vi "Write Standad Header.vi"(8 "error in (no error)":errorcluster, 11 "Save Image in":refnum<class "Save Image.lvclass">) -> (0 "error out":errorcluster, 3 "Save Image out":refnum<class "Save Image.lvclass">)   [LabVIEW 2018, in "Save Image.lvclass"]
uses:
  Save Image.lvclass
  <userlib>/gfitsio/gfitsio-write-key-string.vi
  <userlib>/gfitsio/gfitsio-write-key-integer.vi
  <userlib>/gfitsio/gfitsio-write-key-double.vi
  <userlib>/gfitsio/gfitsio.lvlib
  Simulated_Header/Simulated_Header.lvclass
  <vilib>/Utility/Data Type/NI_Data Type.lvlib
panel:
  out "Header Content":T1
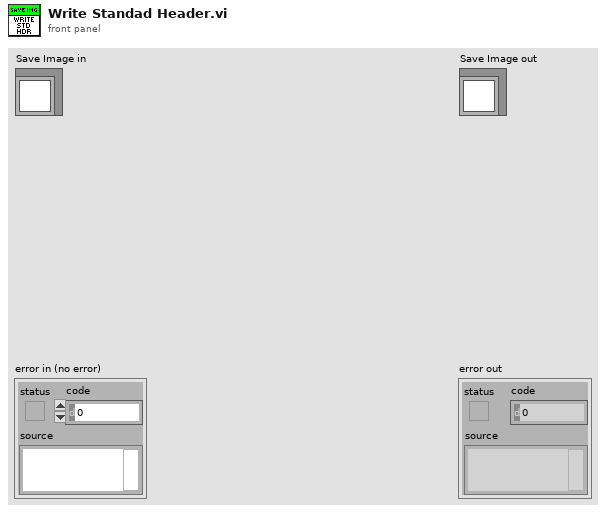
[diagram p1: front panel]
types:
  T1 = cluster{"FILENAME":cluster{"Name":string, "Value":string, "Comment":string}, "OBSERVER":cluster{"Name":string, "Value":string, "Comment":string}, "PROGRID":cluster{"Name":string, "Value":string, "Comment":string}, "OBJECT":cluster{"Name":string, "Value":string, "Comment":string}, "NIGHTDIR":cluster{"Name":string, "Value":string, "Comment":string}, "CHANNEL":cluster{"Name":string, "Value":string, "Comment":string}, "INSTRUME":cluster{"Name":string, "Value":string, "Comment":string}, "NEXPSEQ":cluster{"Name":string, "Value":u16, "Comment":string}, "SEQINDEX":cluster{"Name":string, "Value":u16, "Comment":string}, "OBSTYPE":cluster{"Name":string, "Value":string, "Comment":string}, "READMOD":cluster{"Name":string, "Value":string, "Comment":string}, "READMODE":cluster{"Name":string, "Value":string, "Comment":string}, "ACQMODE":cluster{"Name":string, "Value":string, "Comment":string}, "PREAMP":cluster{"Name":string, "Value":string, "Comment":string}, "READOUT":cluster{"Name":string, "Value":string, "Comment":string}, "VSHIFT":cluster{"Name":string, "Value":string, "Comment":string}, "TRIGGER":cluster{"Name":string, "Value":string, "Comment":string}, "EMMODE":cluster{"Name":string, "Value":string, "Comment":string}, "EMGAIN":cluster{"Name":string, "Value":u16, "Comment":string}, "VBIN":cluster{"Name":string, "Value":u16, "Comment":string}, "HBIN":cluster{"Name":string, "Value":u16, "Comment":string}, "INITLIN":cluster{"Name":string, "Value":u16, "Comment":string}, "INITCOL":cluster{"Name":string, "Value":u16, "Comment":string}, "FINALLIN":cluster{"Name":string, "Value":u16, "Comment":string}, "FINALCOL":cluster{"Name":string, "Value":u16, "Comment":string}, "KSERLEN":cluster{"Name":string, "Value":u16, "Comment":string}, "SHUTTER":cluster{"Name":string, "Value":string, "Comment":string}, "OPENSHT":cluster{"Name":string, "Value":u16, "Comment":string}, "CLOSESHT":cluster{"Name":string, "Value":u16, "Comment":string}, "DATE":cluster{"Name":string, "Value":string, "Comment":string}, "GAIN":cluster{"Name":string, "Value":dbl, "Comment":string}, "GAINERR":cluster{"Name":string, "Value":dbl, "Comment":string}, "RDNOISE":cluster{"Name":string, "Value":dbl, "Comment":string}, "RNOISERR":cluster{"Name":string, "Value":dbl, "Comment":string}, "SKYFIBER":cluster{"Name":string, "Value":string, "Comment":string}, "CALFIBER":cluster{"Name":string, "Value":string, "Comment":string}, "UTDATE":cluster{"Name":string, "Value":string, "Comment":string}, "LOCTIME":cluster{"Name":string, "Value":string, "Comment":string}, "MJD":cluster{"Name":string, "Value":dbl, "Comment":string}, "OBSLON":cluster{"Name":string, "Value":string, "Comment":string}, "OBSLAT":cluster{"Name":string, "Value":string, "Comment":string}, "OBSALT":cluster{"Name":string, "Value":dbl, "Comment":string}, "EXPTIME":cluster{"Name":string, "Value":dbl, "Comment":string}, "TELRA":cluster{"Name":string, "Value":string, "Comment":string}, "TELDEC":cluster{"Name":string, "Value":string, "Comment":string}, "RA":cluster{"Name":string, "Value":string, "Comment":string}, "DEC":cluster{"Name":string, "Value":string, "Comment":string}, "RA_DEG":cluster{"Name":string, "Value":dbl, "Comment":string}, "DEC_DEG":cluster{"Name":string, "Value":dbl, "Comment":string}, "EPOCH":cluster{"Name":string, "Value":dbl, "Comment":string}, "HA":cluster{"Name":string, "Value":string, "Comment":string}, "HAD":cluster{"Name":string, "Value":dbl, "Comment":string}, "AIRMASS":cluster{"Name":string, "Value":dbl, "Comment":string}, "AMSTART":cluster{"Name":string, "Value":dbl, "Comment":string}, "AMEND":cluster{"Name":string, "Value":dbl, "Comment":string}, "XOFFSET":cluster{"Name":string, "Value":dbl, "Comment":string}, "YOFFSET":cluster{"Name":string, "Value":dbl, "Comment":string}, "PA":cluster{"Name":string, "Value":dbl, "Comment":string}, "CAMFOC":cluster{"Name":string, "Value":string, "Comment":string}, "TELFOC":cluster{"Name":string, "Value":dbl, "Comment":string}, "TCSUT":cluster{"Name":string, "Value":string, "Comment":string}, "TCSST":cluster{"Name":string, "Value":string, "Comment":string}, "MOONDIST":cluster{"Name":string, "Value":dbl, "Comment":string}, "MOONALT":cluster{"Name":string, "Value":dbl, "Comment":string}, "MOONPHAS":cluster{"Name":string, "Value":string, "Comment":string}, "ADC":cluster{"Name":string, "Value":string, "Comment":string}, "ADCSPEED":cluster{"Name":string, "Value":dbl, "Comment":string}, "CALMIRR":cluster{"Name":string, "Value":string, "Comment":string}, "GUIDING":cluster{"Name":string, "Value":string, "Comment":string}, "GUIDTEXP":cluster{"Name":string, "Value":dbl, "Comment":string}, "GUIDFREQ":cluster{"Name":string, "Value":dbl, "Comment":string}, "GUIDOBJX":cluster{"Name":string, "Value":dbl, "Comment":string}, "GUIDOBJY":cluster{"Name":string, "Value":dbl, "Comment":string}, "AVGYCORR":cluster{"Name":string, "Value":dbl, "Comment":string}, "AVGXCORR":cluster{"Name":string, "Value":dbl, "Comment":string}, "GFOCUS":cluster{"Name":string, "Value":dbl, "Comment":string}, "THARLAMP":cluster{"Name":string, "Value":string, "Comment":string}, "HALLAMP":cluster{"Name":string, "Value":string, "Comment":string}, "AGITATOR":cluster{"Name":string, "Value":string, "Comment":string}, "THARMIRR":cluster{"Name":string, "Value":string, "Comment":string}, "DSTATUS":cluster{"Name":string, "Value":string, "Comment":string}, "DPOS":cluster{"Name":string, "Value":dbl, "Comment":string}, "DTEMP":cluster{"Name":string, "Value":dbl, "Comment":string}, "DHUM":cluster{"Name":string, "Value":string, "Comment":string}, "DLAMP":cluster{"Name":string, "Value":string, "Comment":string}, "DFLAT":cluster{"Name":string, "Value":string, "Comment":string}, "TEMPEXT":cluster{"Name":string, "Value":string, "Comment":string}, "PRESSURE":cluster{"Name":string, "Value":string, "Comment":string}, "HUMIDITY":cluster{"Name":string, "Value":string, "Comment":string}, "WINDDIR":cluster{"Name":string, "Value":string, "Comment":string}, "WINSPEED":cluster{"Name":string, "Value":dbl, "Comment":string}, "SHTTTL":cluster{"Name":string, "Value":string, "Comment":string}, "COOLER":cluster{"Name":string, "Value":string, "Comment":string}, "TEMP":cluster{"Name":string, "Value":u16, "Comment":string}, "TEMPST":cluster{"Name":string, "Value":string, "Comment":string}, "SERN":cluster{"Name":string, "Value":u16, "Comment":string}, "COMMENT":cluster{"Name":string, "Value":string, "Comment":string}, "SIMPLE":cluster{"Name":string, "Value":string, "Comment":string}, "BITPIX":cluster{"Name":string, "Value":u16, "Comment":string}, "NAXIS":cluster{"Name":string, "Value":u16, "Comment":string}, "EXTEND":cluster{"Name":string, "Value":string, "Comment":string}, "FRAME_T":cluster{"Name":string, "Value":string, "Comment":string}, "VCLOCK":cluster{"Name":string, "Value":string, "Comment":string}, "ADCHNNL":cluster{"Name":string, "Value":u16, "Comment":string}, "JD":cluster{"Name":string, "Value":dbl, "Comment":string}, "SD":cluster{"Name":string, "Value":string, "Comment":string}}
  T2 = cluster{"Name":string, "Value":string, "Comment":string}
  T3 = cluster{"Name":string, "Value":u16, "Comment":string}
  T4 = typedef "NI_Data Type.lvlib/Data Type.ctl" = enum8{"Invalid Type", "Void", "I8", "I16", "I32", "I64", "U8", "U16", "U32", "U64", "Single Float", "Double Float", "Extended Float", "Single Complex", "Double Complex", "Extended Complex", "Enum U8", "Enum U16", "Enum U32", "Enum U64", "Single Float With Unit", "Double Float With Unit", "Extended Float With Unit", "Single Complex with Unit", "Double Complex with Unit", "Extended Complex with Unit", "Boolean", "String", "Path", "Picture", "Tag", "Array", "Cluster", "Variant", "LV Variant", "Waveform", "Timestamp", "Digital Waveform", "Digital Data", "ExpressData", "Refnum", "External Data", "VI", "Poly VI", "LabVIEW Class Instance", "Fixed Point"}
  T5 = cluster{"Name":string, "Value":i32, "Comment":string}
  T6 = cluster{"Name":string, "Value":dbl, "Comment":string}
  T7 = typedef "gfitsio.lvlib/gfitsio-refnum.ctl" = refnum<k1>
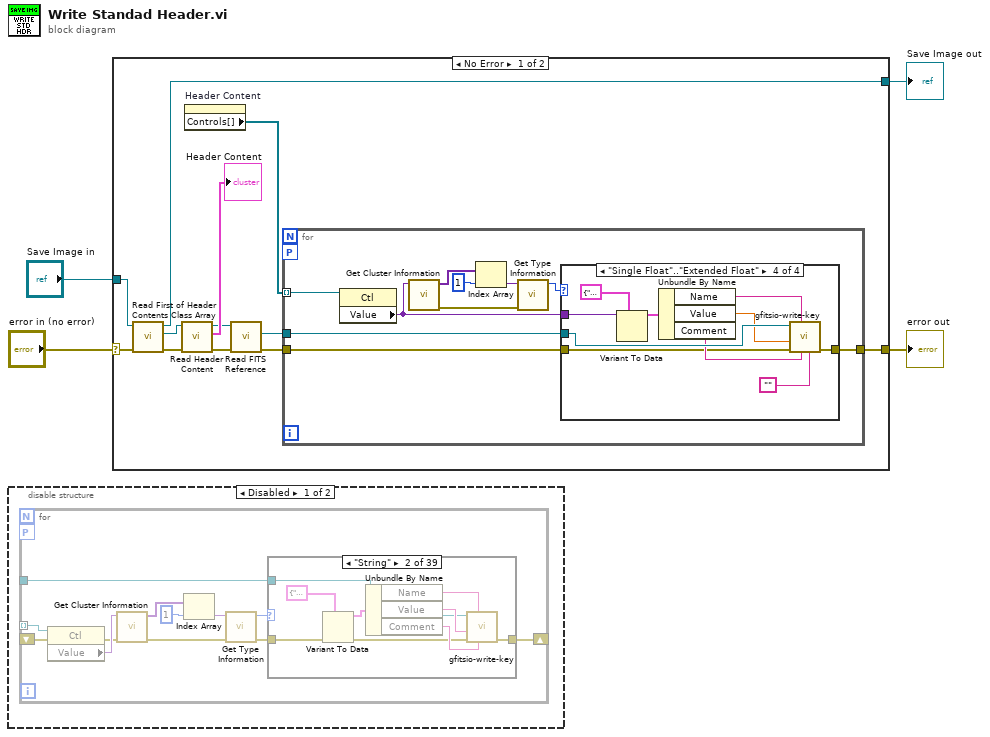
[diagram p0: block diagram]
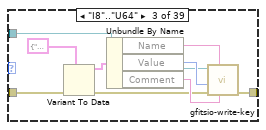
[diagram p3: hidden frame]
diagram:
  n1 = disable-structure shown="Disabled" {
    frame Disabled {
      n2 = for {
        tunnel: _ -> [w16] mode=indexing
        tunnel: _ -> [w5]
        workers-P: _ -> [_]
        shift-right: [w6] -> _
        shift-left: _ -> [w15]
        n3 = property class="Ctl"(reference=w16, error in=w15) -> (error out=w9:errorcluster, "Value"=w12:variant)  [unwired: 1 out]
        n4 = call <vilib>:"Get Cluster Information.vi"("error in (no error)"=w9, "Variant"=w12) -> ("error out"=w8:errorcluster, "Cluster Elements"=w14:variant[])  [unwired: 8 in]
        n5 = Index Array(array=w14, index=1) -> (element=w13:variant)
        n6 = call <vilib>:"Get Type Information.vi"("error in (no error)"=w8, "Variant"=w13) -> ("error out"=w7:errorcluster, "Type"=w10:T4)  [unwired: 5 in, 3 out]
        n7 = case shown="\"String\"" w10 {
          tunnel: w7 -> [w17 w21 w31 _ _ _ _ _ _ _ _ _ _ _ _ _ _ _ _ _ _ _ _ _ _ _ _ _ _ _ _ _ _ _ _ _ _ _ _]
          tunnel: [w17 w19 w29 _ _ _ _ _ _ _ _ _ _ _ _ _ _ _ _ _ _ _ _ _ _ _ _ _ _ _ _ _ _ _ _ _ _ _ _] -> w6
          tunnel: w5 -> [_ w18 w28 _ _ _ _ _ _ _ _ _ _ _ _ _ _ _ _ _ _ _ _ _ _ _ _ _ _ _ _ _ _ _ _ _ _ _ _]
          frame "Invalid Type", Default {
          }
          frame "String" {
            n8 = Variant To Data(error in=w21, type=T2 {"Name"="", "Value"="", "Comment"=""} ("SERN")) -> (data=w23:T2, error out=w20:errorcluster)  [unwired: 1 in]
            n9 = Unbundle By Name(w23) -> ("Name"=w24:string, "Value"=w25:string, "Comment"=w26:string)
            n10 = call-poly <userlib>:"gfitsio-write-key.vi"("comment"=w26, "keyname"=w24, "error in (no error)"=w20, "value"=w25, "gfits refnum"=w18) -> ("error out"=w19:errorcluster)  [unwired: 5 in, 1 out]
          }
          frame "I8".."U64" {
            n11 = Variant To Data(error in=w31, type=T3 {"Name"="", "Value"=0, "Comment"=""} ("SERN")) -> (data=w32:T3, error out=w30:errorcluster)  [unwired: 1 in]
            n12 = Unbundle By Name(w32) -> ("Name"=w33:string, "Value"=w34:u16, "Comment"=w35:string)
            n13 = call-poly <userlib>:"gfitsio-write-key.vi"("comment"=w35, "keyname"=w33, "error in (no error)"=w30, "value"=w34, "gfits refnum"=w28) -> ("error out"=w29:errorcluster)  [unwired: 5 in, 1 out]
          }
          frame "Single Float" {
          }
          frame "Double Float" {
          }
          frame "Extended Float" {
          }
          frame "Single Complex" {
          }
          frame "Double Complex" {
          }
          frame "Extended Complex" {
          }
          frame "Enum U8" {
          }
          frame "Enum U16" {
          }
          frame "Enum U32" {
          }
          frame "Enum U64" {
          }
          frame "Single Float With Unit" {
          }
          frame "Double Float With Unit" {
          }
          frame "Extended Float With Unit" {
          }
          frame "Single Complex with Unit" {
          }
          frame "Double Complex with Unit" {
          }
          frame "Extended Complex with Unit" {
          }
          frame "Boolean" {
          }
          frame "Path" {
          }
          frame "Picture" {
          }
          frame "Tag" {
          }
          frame "Array" {
          }
          frame "Cluster" {
          }
          frame "Variant" {
          }
          frame "LV Variant" {
          }
          frame "Waveform" {
          }
          frame "Timestamp" {
          }
          frame "Digital Waveform" {
          }
          frame "Digital Data" {
          }
          frame "ExpressData" {
          }
          frame "Refnum" {
          }
          frame "External Data" {
          }
          frame "VI" {
          }
          frame "Poly VI" {
          }
          frame "LabVIEW Class Instance" {
          }
          frame "Fixed Point" {
          }
          frame "Void" {
          }
        }
      }
    }
    frame Enabled {
    }
  }
  n14 = case shown="No Error" "error in (no error)" {
    selector: "error in (no error)" -> [w47 w88]
    tunnel: [w38 w88] -> w1
    tunnel: [w45 w89] -> w2
    tunnel: "Save Image in" -> [w46 w89]
    frame No Error {
      n15 = call "Read First of Header Contents Class Array.vi"("error in (no error)"=w47, "Save Image in"=w46) -> ("error out"=w43:errorcluster, "Simulated_Header.lvclass"=w44:refnum<class "Simulated_Header.lvclass">, "Save Image out"=w45:refnum<class "Save Image.lvclass">)  [unwired: 7 in]
      n16 = call "Read Header Content.vi"("error in (no error)"=w43, "Simulated_Header in"=w44) -> ("error out"=w40:errorcluster, "Header Content"=→"Header Content":T1, "Simulated_Header out"=w41:refnum<class "Simulated_Header.lvclass">)  [unwired: 7 in]
      n17 = property on="Header Content" class="Clust (strict)"() -> ("Controls[]"=w36:refnum<vi>[])  [unwired: 2 in, 2 out]
      n18 = call "Read FITS Reference.vi"("error in (no error)"=w40, "Simulated_Header in"=w41) -> ("error out"=w37:errorcluster, "gfits refnum"=w39:T7)  [unwired: 7 in, 1 out]
      n19 = for {
        tunnel: w36 -> [w57] mode=indexing
        tunnel: w39 -> [w56]
        workers-P: _ -> [_]
        tunnel: [w55] -> w38
        tunnel: w37 -> [w49]
        n20 = property class="Ctl"(reference=w57) -> ("Value"=w48:variant)  [unwired: 1 in, 2 out]
        n21 = call <vilib>:"Get Cluster Information.vi"("Variant"=w48) -> ("error out"=w54:errorcluster, "Cluster Elements"=w52:variant[])  [unwired: 9 in]
        n22 = Index Array(array=w52, index=1) -> (element=w51:variant)
        n23 = call <vilib>:"Get Type Information.vi"("error in (no error)"=w54, "Variant"=w51) -> ("Type"=w50:T4)  [unwired: 5 in, 4 out]
        n24 = case shown="\"Single Float\"..\"Extended Float\"" w50 {
          tunnel: w56 -> [_ w67 w77 w87]
          tunnel: [w58 w61 w71 w81] -> w55
          tunnel: w49 -> [w58 w60 w70 w80]
          tunnel: w48 -> [_ w59 w69 w79]
          frame "Invalid Type", Default {
          }
          frame "String" {
            n25 = Variant To Data(type=T2 {"Name"="", "Value"="", "Comment"=""} ("SERN"), Variant=w59) -> (data=w63:T2)  [unwired: 1 in, 1 out]
            n26 = Unbundle By Name(w63) -> ("Name"=w64:string, "Value"=w65:string, "Comment"=w66:string)
            n27 = call-poly <userlib>:"gfitsio-write-key.vi"("comment"=w66, "keyname"=w64, "error in (no error)"=w60, "value"=w65, "gfits refnum"=w67) -> ("error out"=w61:errorcluster)  [unwired: 5 in, 1 out]
          }
          frame "I8".."U64" {
            n28 = Variant To Data(type=T5 {"Name"="", "Value"=0, "Comment"=""} ("SERN"), Variant=w69) -> (data=w73:T5)  [unwired: 1 in, 1 out]
            n29 = Unbundle By Name(w73) -> ("Name"=w74:string, "Value"=w75:i32, "Comment"=w76:string)
            n30 = call-poly <userlib>:"gfitsio-write-key.vi"("units"="", "comment"=w76, "keyname"=w74, "error in (no error)"=w70, "value"=w75, "gfits refnum"=w77) -> ("error out"=w71:errorcluster)  [unwired: 4 in, 1 out]
          }
          frame "Single Float".."Extended Float" {
            n31 = Variant To Data(type=T6 {"Name"="", "Value"=0.0, "Comment"=""} ("SERN"), Variant=w79) -> (data=w83:T6)  [unwired: 1 in, 1 out]
            n32 = Unbundle By Name(w83) -> ("Name"=w84:string, "Value"=w85:dbl, "Comment"=w86:string)
            n33 = call-poly <userlib>:"gfitsio-write-key.vi"("units"="", "comment"=w86, "keyname"=w84, "error in (no error)"=w80, "value"=w85, "gfits refnum"=w87) -> ("error out"=w81:errorcluster)  [unwired: 4 in, 1 out]
          }
        }
      }
    }
    frame Error {
    }
  }
  "error out" <- w1
  "Save Image out" <- w2
